vi "log file-1 MOD.vi"   [LabVIEW 2019]
uses:
  AppData/Local/Temp/Status.vi
types:
  T1 = enum16{"open", "replace", "create", "open or create", "replace or create", "replace or create with confirmation"}
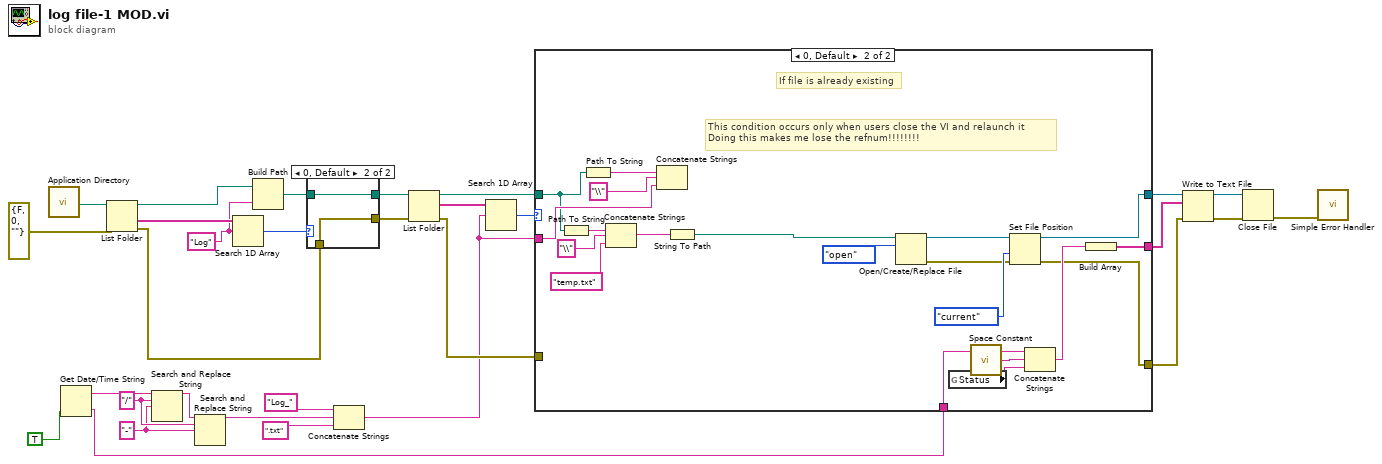
[diagram p0: block diagram]
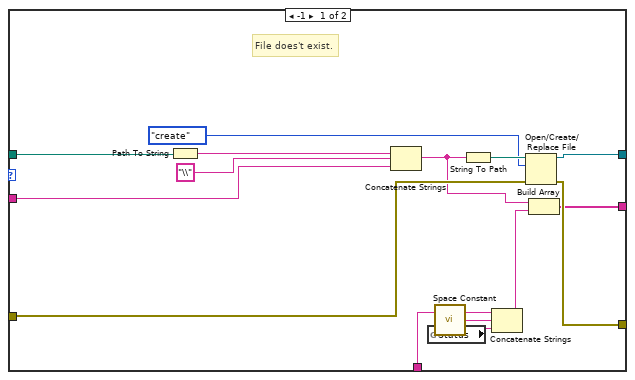
[diagram p2: hidden frame]
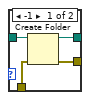
[diagram p3: hidden frame]
diagram:
  w11 = "-" ("chaîne de remplacement (\"\")")
  w13 = "/" ("chaîne recherchée")
  w26 = "Log" ("élément")
  n1 = call <vilib>:"Application Directory.vi"() -> ("Application Directory"=w5:path)
  n2 = Get Date/Time String(want seconds? (F)=TRUE ("secondes ? (F)")) -> (date string=w7:string, time string=w4:string)  [unwired: 2 in]
  n3 = List Folder(path=w5, error in=errorcluster {"status"=FALSE, "code"=0, "source"=""} ("entrée d'erreur")) -> (path out=w28:path, folder names=w30:string[], error out=w19:errorcluster)  [unwired: 2 in, 1 out]
  n4 = Search and Replace String(input string=w7, search string=w13, replace string=w11) -> (result string=w10:string)  [unwired: 5 in, 3 out]
  n5 = Search and Replace String(input string=w10, search string=w13, replace string=w11) -> (result string=w12:string)  [unwired: 5 in, 3 out]
  n6 = Search 1D Array(1D array=w30, element=w26) -> (index of element=w29:i32)  [unwired: 1 in]
  n7 = Build Path(base path=w28, name or relative path=w26) -> (appended path=w27:path)
  n8 = case shown="0, Default" w29 {
    tunnel: [w34 w36] -> w25
    tunnel: w27 -> [w33 w36]
    tunnel: w19 -> [w32 w35]
    tunnel: [w31 w35] -> w18
    frame -1 {
      n9 = Create Folder(path (use dialog)=w33, error in=w32) -> (created path=w34:path, error out=w31:errorcluster)  [unwired: 1 in, 1 out]
    }
    frame 0, Default {
    }
  }
  n10 = Concatenate Strings("Log_" ("chaîne"), w12, ".txt" ("chaîne")) -> (w6:string)
  n11 = List Folder(path=w25, error in=w18) -> (path out=w22:path, filenames=w24:string[], error out=w17:errorcluster)  [unwired: 2 in, 1 out]
  n12 = Search 1D Array(1D array=w24, element=w6) -> (index of element=w23:i32)  [unwired: 1 in]
  n13 = case shown="0, Default" w23 {
    tunnel: w22 -> [w51 w59]
    tunnel: w6 -> [w49 w60]
    tunnel: [w37 w58] -> w21
    tunnel: [w43 w67] -> w2
    tunnel: [w45 w57] -> w1
    tunnel: w17 -> [w44 _]
    tunnel: w4 -> [w38 w71]
    frame -1 {
      # "File does't exist."
      n14 = Path To String(path=w51) -> (string=w50:string)
      n15 = Concatenate Strings(w50, "\\" ("chaîne"), w49) -> (w39:string)
      n16 = global read "Status.vi" "Status"() -> (w42:string)
      n17 = call <vilib>:"Space Constant.vi"() -> ("String"=w41:string)
      n18 = String To Path(string=w39) -> (path=w48:path)
      n19 = Concatenate Strings(w38, w41, w42) -> (w40:string)
      n20 = Open/Create/Replace File(file path (use dialog)=w48, error in=w44, operation (0:open)=T1."create" ("opération (0 : open)")) -> (refnum out=w37:refnum<file>, error out=w45:errorcluster)  [unwired: 3 in, 1 out]
      n21 = Build Array(w39, w40) -> (w43:string[])
    }
    frame 0, Default {
      # "This condition occurs only when users close the VI and relaunch it\nDoing this makes me lose the refnum!!!!!!!!"
      # "If file is already existing"
      n22 = Path To String(path=w59) -> (string=w64:string)
      n23 = Path To String(path=w59) -> (string=w62:string)
      n24 = Concatenate Strings(w64, "\\" ("chaîne"), "temp.txt" ("chaîne")) -> (w56:string)
      n25 = Concatenate Strings(w62, "\\" ("chaîne"), w60) -> ()  [unwired: 1 out]
      n26 = String To Path(string=w56) -> (path=w52:path)
      n27 = Open/Create/Replace File(file path (use dialog)=w52, operation (0:open)=T1."open" ("opération (0 : open)")) -> (refnum out=w54:refnum<file>, error out=w55:errorcluster)  [unwired: 4 in, 1 out]
      n28 = global read "Status.vi" "Status"() -> (w70:string)
      n29 = call <vilib>:"Space Constant.vi"() -> ("String"=w69:string)
      n30 = Set File Position(refnum=w54, from (0:start)=enum16{"start", "end", "current"}."current" ("à partir de (0 : start)"), error in=w55) -> (refnum out=w58:refnum<file>, error out=w57:errorcluster)  [unwired: 1 in]
      n31 = Concatenate Strings(w71, w69, w70) -> (w68:string)
      n32 = Build Array(w68) -> (w67:string[])
    }
  }
  n33 = Write to Text File(file (use dialog)=w21, text=w2, error in=w1) -> (refnum out=w15:refnum<file>, error out=w16:errorcluster)  [unwired: 1 in, 1 out]
  n34 = Close File(refnum=w15, error in=w16) -> (error out=w14:errorcluster)  [unwired: 1 out]
  n35 = call <vilib>:"Simple Error Handler.vi"("error in (no error)"=w14) -> ()  [unwired: 2 in, 7 out]
